vi "Pre Launch Init.vi"(11 "StopEnabledActor in":refnum<class "StopEnabledActor.lvclass">) -> (0 "error out":errorcluster, 3 "StopEnabledActor out":refnum<class "StopEnabledActor.lvclass">)   [LabVIEW 2017, in "StopEnabledActor.lvclass"]
doc: "(<B>Filename</B>: Actor Framework.lvlib:Actor.lvclass:Pre Launch Init.vi)\n\nDefines behavior that occurs after the Launch Nested Actor method is invoked but before the actor's Actor Core method begins running.\n\nBy default, this method does nothing. A descendant class may override it to define behavior."
uses:
  StopEnabledActor.lvclass
  C:/Program Files (x86)/National Instruments/LabVIEW 2017/vi.lib/ActorFramework/Actor/Actor.lvclass
  Stop Event Message.lvclass
  C:/Program Files (x86)/National Instruments/LabVIEW 2017/vi.lib/NI/Event Source Actor/Event Source/Event Source Messages/Event Generated Msg/Event Generated Msg.lvclass
  <vilib>/NI/Event Source Actor/Event Source/Event/Event.lvclass/Event.ctl
  <vilib>/ActorFramework/Actor/Actor.lvclass/Actor.ctl
  <vilib>/ActorFramework/Message Enqueuer/Message Enqueuer.lvclass/Message Enqueuer.ctl
  <vilib>/NI/Event Source Actor/Event Source/Event Source Messages/Register Msg/Register Msg.lvclass/Register Msg.ctl
  <vilib>/ActorFramework/Message Enqueuer/Init from Existing Queue.vi
  <vilib>/ActorFramework/Message Enqueuer/Enqueue.vi
  <vilib>/NI/Event Source Actor/Event Source/Event Source Messages/Register Msg/Register Msg.lvclass
  C:/Program Files (x86)/National Instruments/LabVIEW 2017/vi.lib/ActorFramework/Message/Message.lvclass
  <vilib>/Utility/LVClass/Get LV Class Name.vi
  <resource>/AFDebug/Generate Trace for Message.vi
  <vilib>/ActorFramework/Message Priority Queue/Priority Enqueue.vi
  <vilib>/ActorFramework/Actor/Actor.lvclass
  <vilib>/ActorFramework/Message Enqueuer/Message Enqueuer.lvclass
  <vilib>/NI/Event Source Actor/Event Source/Event/Event.lvclass
  GlobalStopActor/GlobalStopActor.lvclass
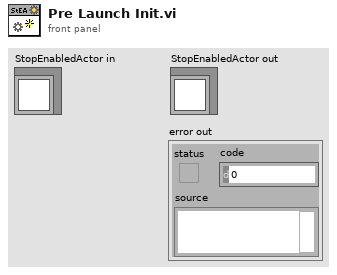
[diagram p1: front panel]
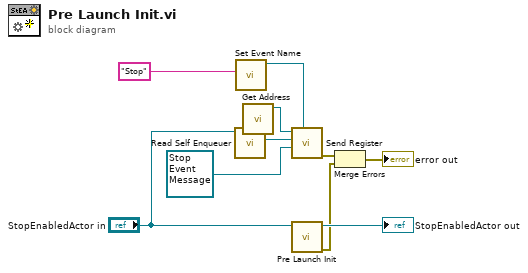
[diagram p0: block diagram]
diagram:
  n1 = call <vilib>:"Read Self Enqueuer.vi"("Actor"="StopEnabledActor in") -> ("Self Enqueuer"=w7:refnum<class "Message Enqueuer.lvclass">)  [unwired: 10 in]
  n2 = call <vilib>:"Set Event Name.vi"("Name (Generic)"="Stop") -> ("Event Out"=w5:refnum<class "Event.lvclass">)  [unwired: 10 in]
  n3 = call "Get Address.vi"() -> ("Enqueuer"=w9:refnum<class "Message Enqueuer.lvclass">)  [unwired: 11 in]
  n4 = call <vilib>:"Send Register.vi"("Event"=w5, "Event Handler"=refnum<class "Stop Event Message.lvclass"> refnum ("Stop Event Message.lvclass"), "Registrant Address"=w7, "Event Source Address"=w9) -> ("Error Out"=w3:errorcluster)  [unwired: 6 in, 1 out]
  n5 = call-parent "Pre Launch Init.vi"("Actor in"="StopEnabledActor in") -> ("error out"=w2:errorcluster, "Actor out"=→"StopEnabledActor out":refnum<class "StopEnabledActor.lvclass">)  [unwired: 9 in]
  n6 = Merge Errors(w3, w2) -> (→"error out":errorcluster)
